vi "Serialize as VTT.vi"(8 "error in (no error)":errorcluster, 11 "Attribute in":refnum<class "Attribute.lvclass">) -> (0 "error out":errorcluster, 2 "VTT Fragment":string, 3 "Attribute out":refnum<class "Attribute.lvclass">)   [LabVIEW 2018, in "VILab.lvlib" / "Attribute.lvclass"]
uses:
  Attribute.lvclass
  Attribute.lvclass/Attribute.ctl
  Data Item.lvclass
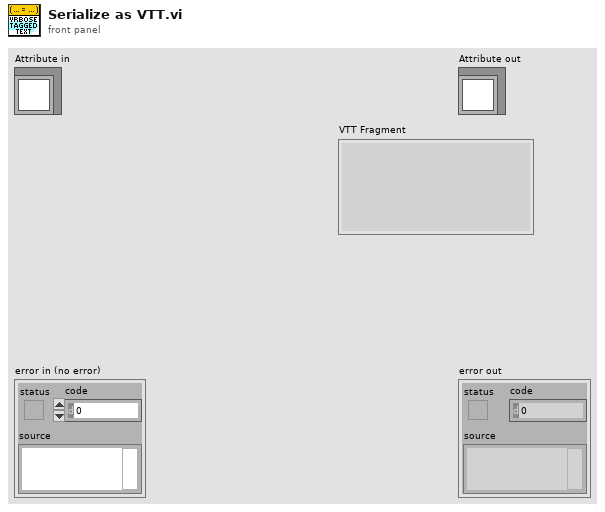
[diagram p1: front panel]
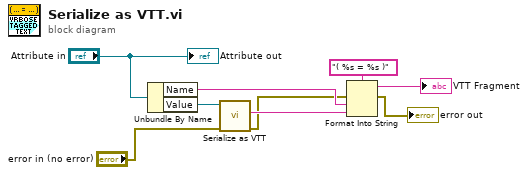
[diagram p0: block diagram]
diagram:
  n1 = Unbundle By Name("Attribute in") -> ("Name"=w5:string, "Value"=w8:refnum<class "Data Item.lvclass">)
  n2 = call-dynamic "Serialize as VTT.vi"("error in (no error)"="error in (no error)", "Data Item in"=w8) -> ("error out"=w2:errorcluster, "VTT Fragment"=w4:string)  [unwired: 7 in, 1 out]
  n3 = Format Into String(format string="( %s = %s )", error in=w2, w5, w4) -> (resulting string=→"VTT Fragment":string, error out=→"error out":errorcluster)  [unwired: 1 in]
  "Attribute out" <- "Attribute in"
